vi "vector_pose_test.vi"() -> ()   [LabVIEW 2011]
uses:
  <vilib>/Analysis/Matrix/Datatypes/RealMatrix.ctl
  <vilib>/Analysis/Matrix/NI_Matrix.lvlib
panel:
  out "RMS mismatch (mm/degree)":dbl
  out "Vector component mismatch":dbl[](array[numeric])
  out "Vector out":dbl[](array[numeric])
  out "Pose":T1
  in  "Vector in":dbl[](array[numeric])
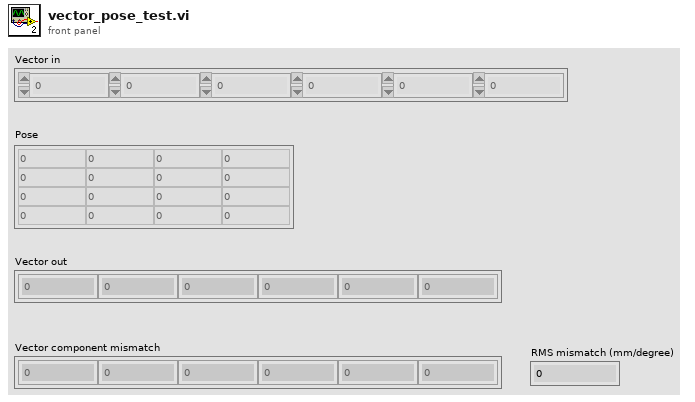
[diagram p1: front panel]
types:
  T1 = typedef "NI_Matrix.lvlib/RealMatrix.ctl" = dbl[][]
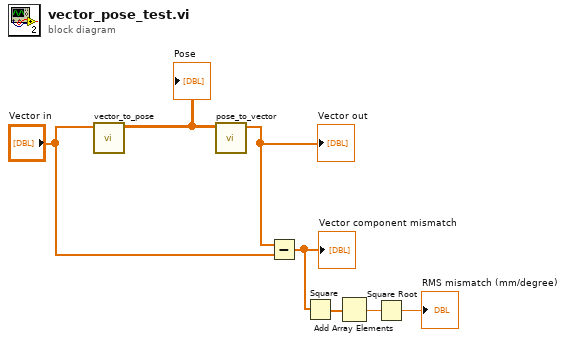
[diagram p0: block diagram]
diagram:
  n1 = call "vector_to_pose.vi"("Pose vector"="Vector in") -> ("Pose"=w3:T1)  [unwired: 10 in]
  "Pose" <- w3
  n2 = call "pose_to_vector.vi"("Pose"=w3) -> ("Pose vector"=w2:dbl[])  [unwired: 10 in]
  "Vector out" <- w2
  n3 = Subtract(x=w2, y="Vector in") -> (x-y=w5:dbl[])
  "Vector component mismatch" <- w5
  n4 = Square(x=w5) -> (x^2=w6:dbl[])
  n5 = Add Array Elements(numeric array=w6) -> (sum=w7:dbl)
  n6 = Square Root(x=w7) -> (sqrt(x)=→"RMS mismatch (mm/degree)":dbl)
